vi "Simple AAV.vi"() -> ()   [LabVIEW 2012]
doc: "This VI acquires, analyzes, and presents data. It is a solution VI to an exercise in the LabVIEW Core I course. Refer to the course manual for instructions."
uses:
  Instance           2 18Saved   Simple AAP .vi
  Instance           3 18Saved   Simple AAP .vi
panel:
  out "Average Value":dbl
  out "Waveform Graph":dynamicdata(graph)
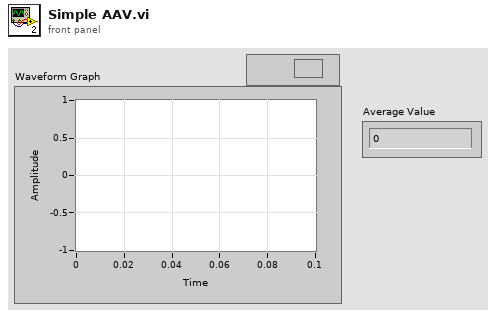
[diagram p1: front panel]
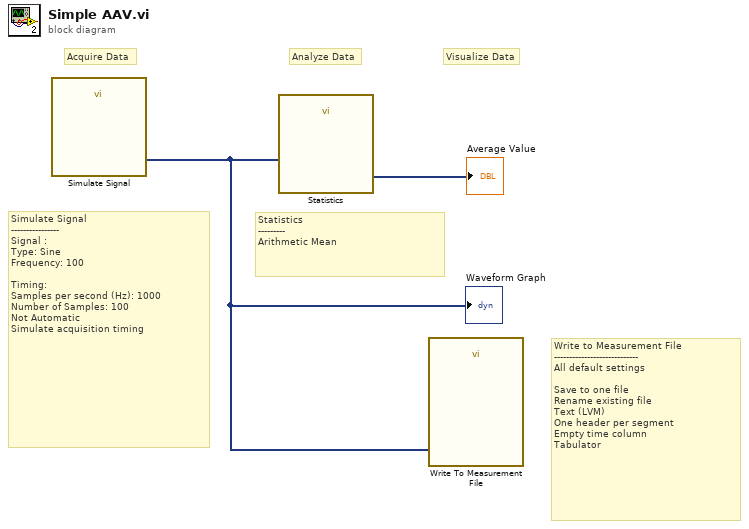
[diagram p0: block diagram]
diagram:
  # "Statistics\n---------\nArithmetic Mean"
  # "Write to Measurement File\n----------------------------\nAll default settings\n\nSave to one file\nRename existing file\nText (LVM)\nOne header per segment\nEmpty time column\nTabulator"
  # "Simulate Signal\n----------------\nSignal :\nType: Sine \nFrequency: 100\n\nTiming:\nSamples per second (Hz): 1000\nNumber of Samples: 100\nNot Automatic\nSimulate acquisition timing"
  # "Visualize Data"
  # "Analyze Data"
  # "Acquire Data"
  n1 = call "Simulate Signal"() -> ("Sine"=w1:dynamicdata)  [unwired: 14 in, 1 out]
  "Waveform Graph" <- w1
  n2 = call "Statistics"("Signals"=w1) -> ("Arithmetic Mean"=→"Average Value":dynamicdata)  [unwired: 25 in, 1 out]
  n3 = call "Write To Measurement File"("Signals"=w1) -> ()  [unwired: 8 in, 3 out]
